vi "Force Close All Instances.vi"(8 "error in (no error)":errorcluster, 11 "Waveform Log in":refnum<class "Waveform Log.lvclass">) -> (0 "error out":errorcluster)   [LabVIEW 2015, in "Waveform Log.lvclass"]
uses:
  Waveform Log.lvclass
  Waveform Log.lvclass/Waveform Log.ctl
  Logs/Segmented Logs/Segmented Log/Segmented Log.lvclass
  Logs/Segmented Logs/Segmented Log/Segmented Log.lvclass/Segmented Log.ctl
  Logs/Log Files/Log File/Log File.lvclass/Log File.ctl
  Logs/Log Files/TDMS Log File/TDMS Log File.lvclass/TDMS Log File.ctl
  Logs/Log Files/Text Log File/Text Log File.lvclass/Text Log File.ctl
  Logs/Segmented Logs/Segmented Log/Close Log File Instance.vi
  Logs/Log Files/Log File/Close Log File.vi
  Logs/Segmented Logs/Segmented Log/Make File Read-Only.vi
  Logs/Segmented Logs/Segmented Log/On Segmented Log Complete.vi
  Logs/Segmented Logs/Segmented Log/On File Close.vi
  Logs/Log Files/TDMS Log File/Close TDMS Log File.vi
  Logs/Log Files/Text Log File/Close Text Log File.vi
  Logs/Log Files/Log File/Log File.lvclass
  Logs/Log Files/TDMS Log File/TDMS Log File.lvclass
  Logs/Log Files/Text Log File/Text Log File.lvclass
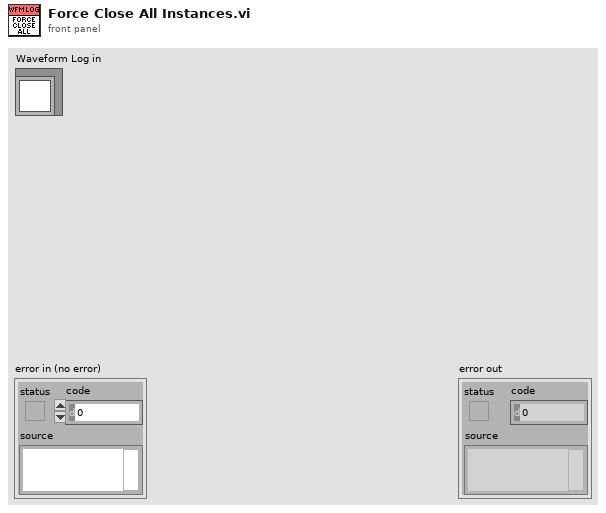
[diagram p1: front panel]
types:
  T1 = typedef "Waveform Log.lvclass/Log Instance.ctl" = cluster{"Segmented Log":refnum<data-value>, "Log Waveforms":T2[], "Log Start":timestamp, "Log Stop":timestamp, "Start Trigger Time":timestamp, "Stop Trigger Time":timestamp, "Time of Last Write":timestamp, "Timeout":dbl, "Stop cmd received":bool}
  T2 = typedef "Waveform Log.lvclass/Log Instance Waveform.ctl" = cluster{"Wfm Info":T3, "Count / Instance":i32, "Previous Segment":u64, "Wfm Complete?":bool, "Last Sample Logged":timestamp, "Data Logged":bool, "Log segmented":bool}
  T3 = typedef "Waveform Log.lvclass/Waveform Information.ctl" = cluster{"Name":string, "Wfm Data Type":T4, "Decimation":u32}
  T4 = typedef "Waveform Log.lvclass/Waveform Data Type.ctl" = enum16{"Double", "ComplexDouble"}
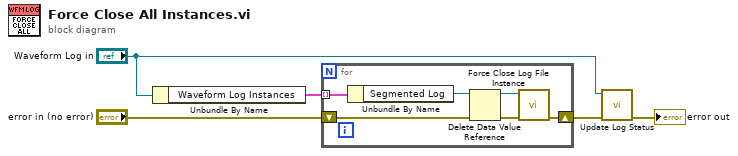
[diagram p0: block diagram]
diagram:
  n1 = Unbundle By Name("Waveform Log in") -> ("Waveform Log Instances"=w4:T1[])
  n2 = for {
    shift-right: [w6] -> w2
    shift-left: "error in (no error)" -> [w10]
    tunnel: w4 -> [w11] mode=indexing
    n3 = Unbundle By Name(w11) -> ("Segmented Log"=w9:refnum<data-value>)
    n4 = Delete Data Value Reference(data value reference=w9, error in=w10) -> (data value=w8:refnum<class "Segmented Log.lvclass">, error out=w7:errorcluster)
    n5 = call "Force Close Log File Instance.vi"("error in (no error)"=w7, "Segmented Log in"=w8) -> ("error out"=w6:errorcluster)  [unwired: 7 in, 2 out]
  }
  n6 = call "Update Log Status.vi"("error in (no error)"=w2, "Waveform Log in"="Waveform Log in") -> ("error out"=→"error out":errorcluster)  [unwired: 8 in, 1 out]
